vi "binary search3VI_Test_as_VI_test.vi"() -> ()   [LabVIEW 2019]
uses:
  <vilib>/Utility/file.llb/Read Delimited Spreadsheet (DBL).vi
panel:
  out "XY Graph":cluster{dbl[], dbl[]}(graph)
  out "Waveform Graph":waveform(dbl)(graph)={"t0"=timestamp(0 s since 1904-01-01), "dt"=0.023255813866853714, "Y"=[0.0, 0.0, 0.00016623700503259897, 0.0004462969955056906, 0.0008978309924714267, 0.0015961199533194304, 0.0026342500932514668, 0.004121169913560152, 0.0061773499473929405, 0.008928230032324791, 0.012496000155806541, 0.016990400850772858, 0.022500399500131607, 0.0290863998234272, 0.03677539899945259, 0.04555860161781311, 0.05539190024137497, 0.0661993995308876, 0.07787880301475525, 0.0903078019618988, 0.10335200279951096, 0.11687199771404266, 0.130731001496315, 0.14479699730873108, 0.158952996134758, 0.1730940043926239, 0.18713100254535675, 0.20099399983882904, 0.21462899446487427, 0.22799499332904816, 0.2410700023174286, 0.25383999943733215, 0.26630398631095886, 0.27847200632095337, 0.2903589904308319, 0.30198800563812256, 0.3133859932422638, 0.32458600401878357, 0.33562299609184265, 0.34653499722480774, 0.3573629856109619, 0.3681490123271942, 0.3789370059967041, 0.38977301120758057, 0.4007050096988678, 0.41178199648857117, 0.4230549931526184, 0.434578001499176, 0.44640401005744934, 0.45859000086784363, 0.47119298577308655, 0.4842720031738281, 0.4978860020637512, 0.5120940208435059, 0.5269529819488525, 0.5425170063972473, 0.5588369965553284, 0.575954020023346, 0.5938990116119385, 0.6126909852027893, 0.6323310136795044, 0.6527979969978333, 0.6740450263023376, 0.6959949731826782, 0.7185379862785339, 0.7415289878845215, 0.7647849917411804, 0.7880899906158447, 0.8111960291862488, 0.8338289856910706, 0.8557040095329285, 0.8765339851379395, 0.8960469961166382, 0.9140009880065918, 0.9301999807357788, 0.9445090293884277, 0.9568610191345215, 0.9672639966011047, 0.9757949709892273, 0.9825940132141113, 0.9878519773483276, 0.9917870163917542, 0.9946330189704895, 0.9966170191764832, 0.9979479908943176, 0.9988049864768982, 0.9993330240249634, 0.9996439814567566, 0.9998189806938171, 0.9999129772186279, 0.9999600052833557, 0.999983012676239, 0.9999930262565613, 0.9999970197677612, 0.9999989867210388, 1.0, 1.0, 1.0, 1.0, 1.0, 1.0, 1.0, 1.0, 1.0, 1.0, 1.0, 1.0, 1.0, 1.0, 1.0, 1.0, 1.0, 1.0, 1.0, 1.0, 1.0, 1.0, 1.0, 1.0, 1.0, 1.0, 1.0, 1.0, 1.0, 1.0, 1.0, 1.0, 1.0, 1.0]}
  in  "RG factor":dbl=1.0
  out "size(s) 2":i32=256
  out "Array":sgl[](array[numeric])=[0.0, 0.0, 0.0, 0.000166237, 0.000446297, 0.000897831, 0.00159612, 0.00263425, 0.00412117, 0.00617735, 0.00892823, 0.012496, 0.0169904, 0.0225004, 0.0290864, 0.0367754, 0.0455586, 0.0553919, 0.0661994, 0.0778788, 0.0903078, 0.103352, 0.116872, 0.130731, 0.144797, 0.158953, 0.173094, 0.187131, 0.200994, 0.214629, 0.227995, 0.24107, 0.25384, 0.266304, 0.278472, 0.290359, 0.301988, 0.313386, 0.324586, 0.335623, 0.346535, 0.357363, 0.368149, 0.378937, 0.389773, 0.400705, 0.411782, 0.423055, 0.434578, 0.446404, 0.45859, 0.471193, 0.484272, 0.497886, 0.512094, 0.526953, 0.542517, 0.558837, 0.575954, 0.593899, 0.612691, 0.632331, 0.652798, 0.674045, 0.695995, 0.718538, 0.741529, 0.764785, 0.78809, 0.811196, 0.833829, 0.855704, 0.876534, 0.896047, 0.914001, 0.9302, 0.944509, 0.956861, 0.967264, 0.975795, 0.982594, 0.987852, 0.991787, 0.994633, 0.996617, 0.997948, 0.998805, 0.999333, 0.999644, 0.999819, 0.999913, 0.99996, 0.999983, 0.999993, 0.999997, 0.999999, 1.0, 1.0, 1.0, 1.0, 1.0, 1.0, 1.0, 1.0, 1.0, 1.0, 1.0, 1.0, 1.0, 1.0, 1.0, 1.0, 1.0, 1.0, 1.0, 1.0, 1.0, 1.0, 1.0, 1.0, 1.0, 1.0, 1.0, 1.0, 1.0, 1.0, 1.0, 1.0, 1.0, 1.0, 0.0, 0.0, 0.0, 0.0, 0.0, 0.0, 0.0, 0.0, 0.0, 0.0, 0.0, 0.0, 0.0, 0.0, 0.0, 0.0, 0.0, 0.0, 0.0, 0.0, 0.0, 0.0, 0.0, 0.0, 0.0, 0.0, 0.0, 0.0, 0.0, 0.0, 0.0, 0.0, 0.0, 0.0, 0.0, 0.0, 0.0, 0.0, 0.0, 0.0, 0.0, 0.0, 0.0, 0.0, 0.0, 0.0, 0.0, 0.0, 0.0, 0.0, 0.0, 0.0, 0.0, 0.0, 0.0, 0.0, 0.0, 0.0, 0.0, 0.0, 0.0, 0.0, 0.0, 0.0, 0.0, 0.0, 0.0, 0.0, 0.0, 0.0, 0.0, 0.0, 0.0, 0.0, 0.0, 0.0, 0.0, 0.0, 0.0, 0.0, 0.0, 0.0, 0.0, 0.0, 0.0, 0.0, 0.0, 0.0, 0.0, 0.0, 0.0, 0.0, 0.0, 0.0, 0.0, 0.0, 0.0, 0.0, 0.0, 0.0, 0.0, 0.0, 0.0, 0.0, 0.0, 0.0, 0.0, 0.0, 0.0, 0.0, 0.0, 0.0, 0.0, 0.0, 0.0, 0.0, 0.0, 0.0, 0.0, 0.0, 0.0, 0.0, 0.0, 0.0, 0.0, 0.0] format="%.6f"
  out "Init Data Out":sgl[](array[numeric])=[0.0, 0.0, 0.000166237, 0.000446297, 0.000897831, 0.00159612, 0.00263425, 0.00412117, 0.00617735, 0.00892823, 0.012496, 0.0169904, 0.0225004, 0.0290864, 0.0367754, 0.0455586, 0.0553919, 0.0661994, 0.0778788, 0.0903078, 0.103352, 0.116872, 0.130731, 0.144797, 0.158953, 0.173094, 0.187131, 0.200994, 0.214629, 0.227995, 0.24107, 0.25384, 0.266304, 0.278472, 0.290359, 0.301988, 0.313386, 0.324586, 0.335623, 0.346535, 0.357363, 0.368149, 0.378937, 0.389773, 0.400705, 0.411782, 0.423055, 0.434578, 0.446404, 0.45859, 0.471193, 0.484272, 0.497886, 0.512094, 0.526953, 0.542517, 0.558837, 0.575954, 0.593899, 0.612691, 0.632331, 0.652798, 0.674045, 0.695995, 0.718538, 0.741529, 0.764785, 0.78809, 0.811196, 0.833829, 0.855704, 0.876534, 0.896047, 0.914001, 0.9302, 0.944509, 0.956861, 0.967264, 0.975795, 0.982594, 0.987852, 0.991787, 0.994633, 0.996617, 0.997948, 0.998805, 0.999333, 0.999644, 0.999819, 0.999913, 0.99996, 0.999983, 0.999993, 0.999997, 0.999999, 1.0, 1.0, 1.0, 1.0, 1.0, 1.0, 1.0, 1.0, 1.0, 1.0, 1.0, 1.0, 1.0, 1.0, 1.0, 1.0, 1.0, 1.0, 1.0, 1.0, 1.0, 1.0, 1.0, 1.0, 1.0, 1.0, 1.0, 1.0, 1.0, 1.0, 1.0, 1.0, 1.0, 1.0]
  out "Time_delay":dbl=0.0020034000044688582
  out "Waveform Chart":sgl[](graph)=[0.62142044, 0.72001696, 0.20885716, -0.5753926, -0.38230708, 0.58657235, -0.3477376, -0.582911, -0.651857, 0.6283151, 0.5730913, 0.36173972, 0.5207331, -0.48867276, 0.15210612, 0.6890529, 0.5306942, -0.26378143, 0.49074304, -0.057357714, 0.38430822, 0.7421285, -0.6798329, 0.34763557, -0.44126472, 0.66128945, -0.24832015, 0.24735387, 0.37451768, 0.4054487, 0.00046555675, 0.6856923, -0.34365377, -0.8148198, 0.81512564, 0.784244, 0.8319391, 0.26890427, 0.75024885, 0.43840554, 0.18249755, 0.44947964, 0.5757427, 0.41672057, 0.035923973, 0.3092466, -0.07364922, 0.116820276, -0.5537282, 0.31966853, -0.57563573, 0.5896217, -0.27219185, 0.055822775, 0.67406166, 0.47628766, 0.62542784, 0.8437422, 0.064215675, 0.01589593, -0.26278058, 0.2836846, -0.35384196, 0.044506878, 0.68132406, 0.54300183, 0.5907837, 0.2485031, 0.3527376, -0.21711658, 0.13470717, 0.51719457, -0.2822412, -0.21560419, -0.62143856, 0.13103122, 0.781316, 0.16840522, 0.58284795, 0.67086715, 0.064738385, -0.021301556, 0.56148136, 0.6931487, -0.46505186, 0.56921506, -0.43838742, -0.19009529, 0.69052017, -0.4208888, 0.47433645, 0.017850956, 0.01586592, 0.65438217, 0.41377568, -0.14761412, -0.75319594, -0.5731791, 0.28266734, -0.5625221, 0.73552287, -0.11405211, -0.17017682, 0.51450074, 0.4409039, -0.5427561, 0.700557, 0.0021174846, -0.29620975, -0.20442839, -0.6257302, -0.017994367, 0.17820944, 0.47936827, 0.30935714, 0.7974526, -0.23194648, -0.48719966, -0.10732513, 0.2547426, 0.49810132, 0.14716087, 0.023656217, -0.04084784, -0.6231085, 0.8863027, 0.60467285, -0.49590448, -0.024021849, -0.16521649, -0.420558, -0.61144716, -0.22350591, -0.53376955, 0.34270176, -0.15217097, 0.07650564, -0.24422438, 0.4192762, -0.5451654, -0.55348283, -0.34254405, 0.53973997, 0.098903336, 0.15355557, 0.71787107, -0.19097427, -0.24973595, -0.44423056, 0.31662533, 0.16389857, -0.24400839, -0.31381682, -0.5660442, 0.04329204, -0.43044645, 0.330074, 0.23989779, 0.8558115, 0.26049945, 0.15877561, 0.5510473, 0.34097514, 0.11767771, 0.26768565, 0.79968506, 0.7292263, 0.18388516, -0.37523308, -0.4819311, 0.1732428, 0.6279844, 0.17108716, -0.032732304, 0.34930098, -0.57931674, 0.48747838, -0.08146755, 0.46578044, 0.5113492, 0.45812106, -0.47813705, 0.19343685, -0.2444466, 0.7540186, 0.7164582, 0.14319786, 0.53713024, 0.50586855, -0.105757736, 0.13849105, -0.41287017, 0.382735, 0.40560797, 0.3698187, 0.46507394, 0.2395662, 0.32460266, 0.4419064, 0.08249853, -0.44895884, 0.691823, 0.43279502, 0.5553753, -0.41031358, -0.025204053, -0.041483756, 0.18711941, 0.533495, 0.6140357, 0.10057529, 0.10789915, -0.19447099, 0.04909005, 0.1724128, -0.25399193, -0.33259284, 0.7255678, -0.30039605, -0.45354944, -0.10721463, -0.41583163, -0.39942315, -0.3095516, 0.50055075, -0.14409436, 0.6157717, 0.5781689, 0.10835169, 0.0023106623, -0.8068952, -0.15795527, 0.15227489, -0.30057448, 0.05099563, -0.07791328, 0.5536137, 0.16933069, -0.61272466, 0.33908916, -0.3173198, -0.6602512, 0.60596067, 0.3896042, 0.77764434, 0.14732972, -0.3821757, 0.5972043, 0.09184901, -0.48094788, -0.096387066, -0.17370601, -0.23523764, 0.3533304, 0.8602584]
  in  "Cold":path=path "C:/Users/Diffusivity/OneDrive - sfu.ca/Mpemba/InvMpemba/cum for InvMP/T3.00.txt"
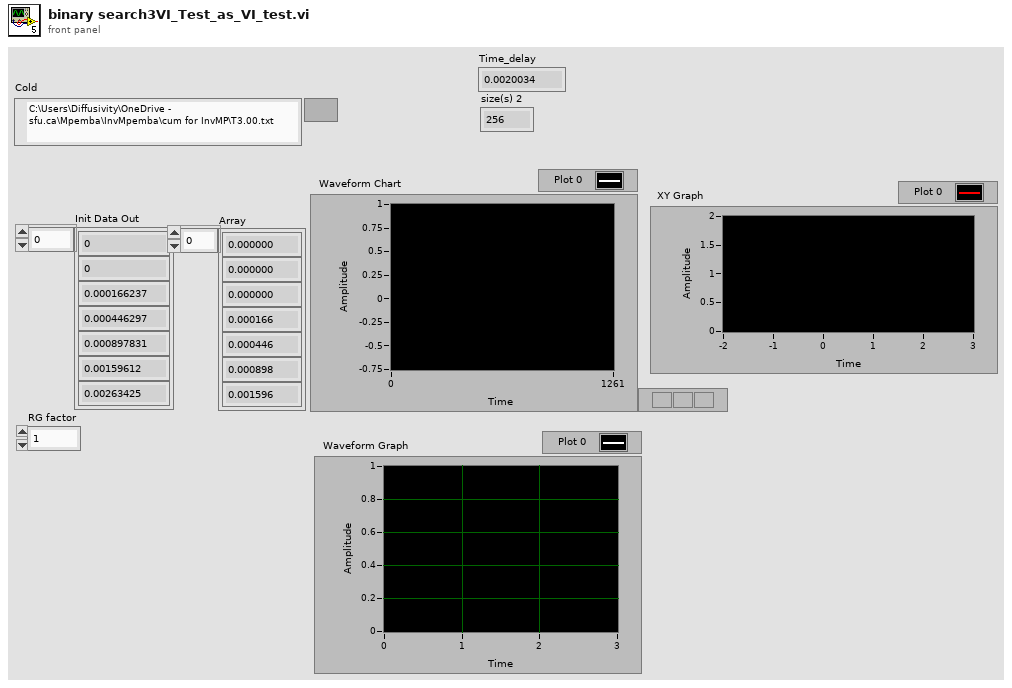
[diagram p1: front panel]
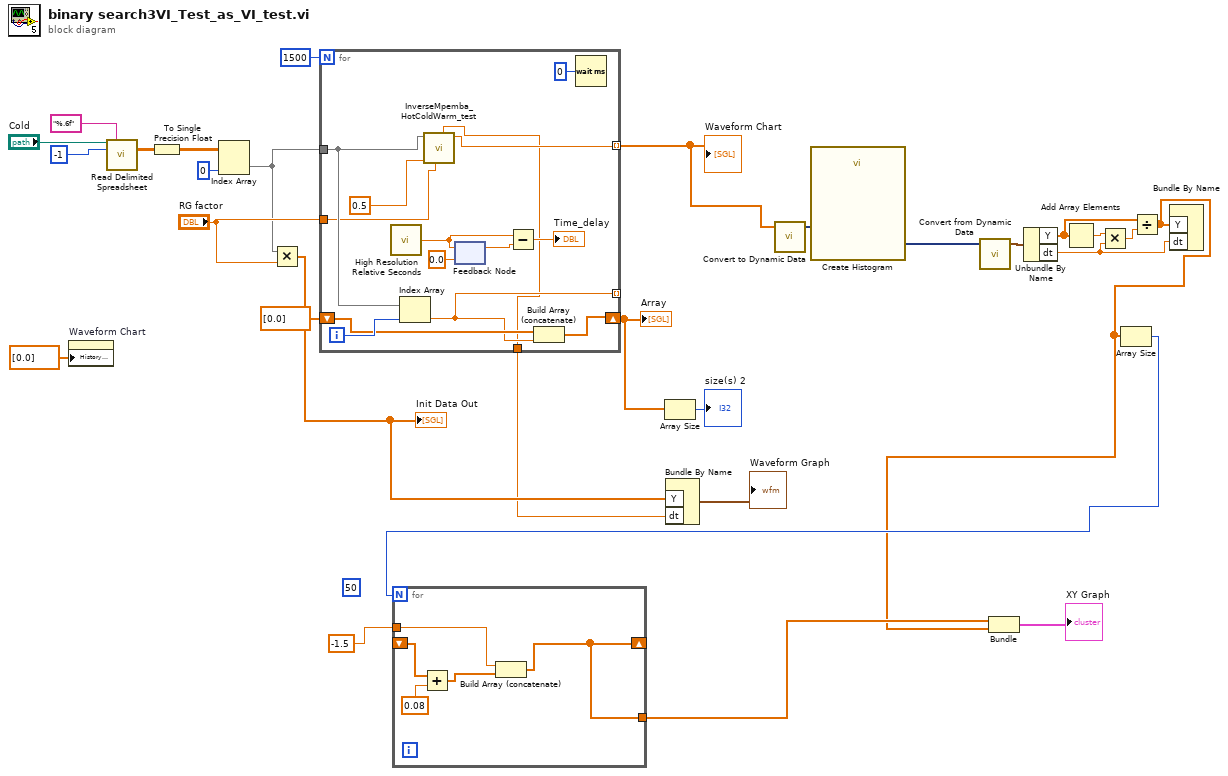
[diagram p0: block diagram]
diagram:
  (unwired) 50
  n1 = property on="Waveform Chart" class="WFChart (strict)"("History Data"=dbl[] [0.0]) -> ()  [unwired: 2 in, 2 out]
  n2 = call-poly <vilib>:"Read Delimited Spreadsheet.vi"("file path (dialog if empty)"="Cold", "format (%.3f)"="%.6f", "number of rows (all:-1)"=-1) -> ("all rows"=w22:dbl[][])  [unwired: 7 in, 5 out]
  n3 = To Single Precision Float(number=w22) -> (single precision float=w25:sgl[][])
  n4 = Index Array(array=w25, index (col)=0 ("disabled index (col)")) -> (element=w7:sgl[])  [unwired: 1 in]
  n5 = Multiply(x=w7, y="RG factor") -> (x*y=w17:dbl[])
  "Init Data Out" <- w17
  n6 = for {
    N: 1500 -> [_]
    tunnel: w7 -> [w34]
    tunnel: [w31] -> w14 mode=indexing
    shift-right: [w37] -> w20
    shift-left: sgl[] [0.0] -> [w38]
    tunnel: [w36] -> _ mode=indexing
    tunnel: "RG factor" -> [w32]
    tunnel: [w30] -> w16
    i -> [w39]
    n7 = call <vilib>:"High Resolution Relative Seconds.vi"() -> ("relative seconds"=w42:dbl)
    n8 = Index Array(array=w34, index=w39) -> (element=w36:sgl)
    n9 = call "InverseMpemba_HotColdWarm_test.vi"("RN"=w32, "X0"=sgl 0.5, "array"=w34) -> ("Xpot"=w31:sgl, "dx"=w30:sgl)  [unwired: 7 in]
    n10 = feedback-in #1(w42) -> ()
    n11 = feedback #1(0.0 ("relative seconds")) -> (w41:dbl)
    n12 = Subtract(x=w42, y=w41) -> (x-y=→"Time_delay":dbl)
    n13 = Build Array (concatenate)(w38, w36) -> (w37:sgl[])
    n14 = Wait (ms)(milliseconds to wait=u32 0) -> ()  [unwired: 1 out]
  }
  "Waveform Chart" <- w14
  "Array" <- w20
  n15 = Array Size(array=w20) -> (size(s)=→"size(s) 2":i32)
  n16 = Bundle By Name("Y"=w17, "dt"=w16) -> (→"Waveform Graph":waveform(dbl))  [unwired: 1 in]
  n17 = call "Convert to Dynamic Data"("Array"=w14) -> ("Dynamic Data Type"=w18:dynamicdata)  [unwired: 3 in]
  n18 = call "Create Histogram"("Signal"=w18) -> ("Histogram"=w13:dynamicdata)  [unwired: 9 in, 1 out]
  n19 = call "Convert from Dynamic Data"("Dynamic Data Type"=w13) -> ("Waveform"=w12:waveform(dbl))  [unwired: 3 in]
  n20 = Unbundle By Name(w12) -> ("Y"=w10:dbl[], "dt"=w8:dbl)
  n21 = Add Array Elements(numeric array=w10) -> (sum=w11:dbl)
  n22 = Multiply(x=w11, y=w8) -> (x*y=w9:dbl)
  n23 = Divide(x=w10, y=w9) -> (x/y=w2:dbl[])
  n24 = Array Size(array=w2) -> (size(s)=w4:i32)
  n25 = for {
    N: w4 -> [_]
    shift-right: [w44] -> _
    shift-left: _ -> [w46]
    tunnel: -1.5 ("Numeric") -> [w47]
    tunnel: [w44] -> w3
    n26 = Add(x=w46, y=0.08 ("Numeric")) -> (x+y=w45:dbl[])
    n27 = Build Array (concatenate)(w47, w45) -> (w44:dbl[])
  }
  n28 = Bundle(w3, w2) -> (→"XY Graph":cluster{dbl[], dbl[]})  [unwired: 1 in]
  n29 = Bundle By Name("Y"=w2, "dt"=w8) -> ()  [unwired: 1 in, 1 out]
